vi "FlexUIActorMaker.vi"(8 "error in (no error)":errorcluster, 10 "UIClassDestination":path, 11 "UIClassName":string) -> (0 "error out":errorcluster, 3 "FlexUIActorMaker.lvlib:FlexUIActorMaker.lvclass":refnum<class "FlexUIActorMaker.lvclass">)   [LabVIEW 2016, in "FlexUIActorMaker.lvlib" / "FlexUIActorMaker.lvclass"]
uses:
  FlexUIActorMaker.lvclass
  FlexUIActorMaker.lvclass/FlexUIActorMaker.ctl
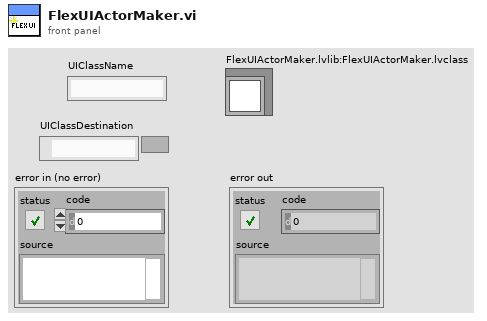
[diagram p1: front panel]
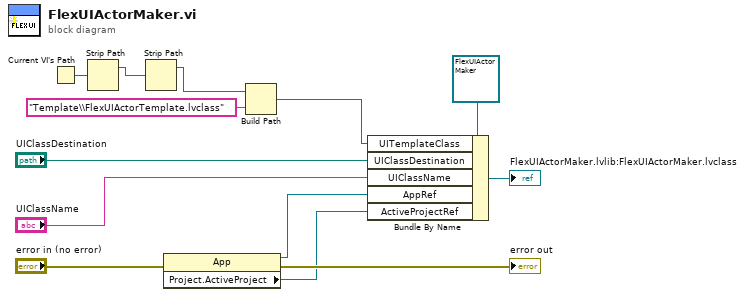
[diagram p0: block diagram]
diagram:
  n1 = Current VI's Path() -> (path=w5:path)
  n2 = Strip Path(path=w5) -> (stripped path=w2:path)  [unwired: 1 out]
  n3 = Strip Path(path=w2) -> (stripped path=w1:path)  [unwired: 1 out]
  n4 = property class="App"(error in="error in (no error)") -> (reference out=w7:refnum<vi>, error out=→"error out":errorcluster, "Project.ActiveProject"=w6:refnum<vi>)  [unwired: 1 in]
  n5 = Build Path(base path=w1, name or relative path="Template\\FlexUIActorTemplate.lvclass") -> (appended path=w3:path)
  n6 = Bundle By Name(cluster=refnum<class "FlexUIActorMaker.lvclass"> refnum ("FlexUIActorMaker.lvlib:FlexUIActorMaker.lvclass"), "UITemplateClass"=w3, "UIClassDestination"="UIClassDestination", "UIClassName"="UIClassName", "AppRef"=w7, "ActiveProjectRef"=w6) -> (→"FlexUIActorMaker.lvlib:FlexUIActorMaker.lvclass":refnum<class "FlexUIActorMaker.lvclass">)
